vi "PH_uOPA_DelayController.PC Get data.vi"(0 "i ref in":refnum<vi>, 5 "error IO":errorcluster) -> (14 "i ref out":refnum<vi>, 19 "error out":errorcluster)   [LabVIEW 2014, in "PH_uOPA_DelayController.lvlib"]
doc: "This is the proc case \"Get Data\": It communicates with hardware to get data and writes them to own attributes."
uses:
  PH_uOPA_DelayController.lvlib
  PH_Basics/PH_StatusHandler/PH_StatusHandler.Status.ctl
  PH_Devices/PH_TKTDS-30xx/PH_TKTDS-30xx.Waveform to fetch.ctl
  PH_Devices/PH_TKTDS-30xx/PH_TKTDS-30xx.Waveform Limits.ctl
  PH_Devices/PH_TKTDS-30xx/PH_TKTDS-30xx.lvlib
  PH_Basics/PH_StatusHandler/PH_StatusHandler.lvlib
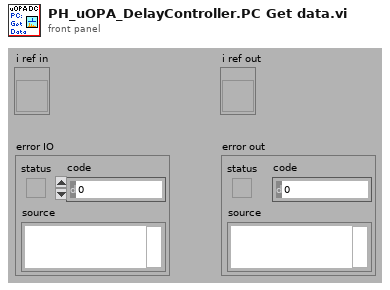
[diagram p1: front panel]
types:
  T1 = typedef "PH_StatusHandler.lvlib/PH_StatusHandler.Status.ctl" = i16
  T2 = typedef "PH_TKTDS-30xx.lvlib/PH_TKTDS-30xx.i attribute.ctl" = cluster{"Default VISA Resource":string, "VISA Resource Name":refnum<visa-resource-name>, "Revision":cluster{"Instrument Driver":string, "Instrument Firmware":string}, "Selftest":cluster{"Result":u32, "Message":string}, "Channels":T3[], "Trigger Configuration":T5, "Acquisition Configuration":T6, "Fetched Waveforms":T7[], "GUI Refs":T8, "State":T1, "Error Message":string, "Allow Prdc Loop?":bool}
  T3 = typedef "PH_TKTDS-30xx.lvlib/PH_TKTDS-30xx.Channel Config.ctl" = cluster{"Channel Name":string, "Input Impedance":string, "Max Input Frequency":string, "Vertical Coupling":i32, "Channel Enabled":bool, "Probe Attenuation":dbl, "Vertical Range":dbl, "Vertical Offset":dbl, "Waveform Limits":T4}
  T4 = typedef "PH_TKTDS-30xx.lvlib/PH_TKTDS-30xx.Waveform Limits.ctl" = cluster{"Start":i32, "End":i32}
  T5 = typedef "PH_TKTDS-30xx.lvlib/PH_TKTDS-30xx.Trigger Config.ctl" = cluster{"Source":string, "Slope":i32, "Level [V]":dbl}
  T6 = typedef "PH_TKTDS-30xx.lvlib/PH_TKTDS-30xx.Acquisition Config.ctl" = cluster{"Time base":dbl, "Record Length":u16, "Start Time":dbl, "Type":i32, "Continuous":bool}
  T7 = typedef "PH_TKTDS-30xx.lvlib/PH_TKTDS-30xx.fetched Waveform.ctl" = cluster{"Source":string, "Actual Points":u32, "Initial X":dbl, "X Increment":dbl, "Waveform Array":dbl[]}
  T8 = typedef "PH_TKTDS-30xx.lvlib/PH_TKTDS-30xx.GUI Refs.ctl" = cluster{"Trigger":refnum<vi>, "Acquisition":refnum<vi>, "State":refnum<vi>, "Delete":refnum<vi>, "Channel to be positioned":refnum<vi>, "Postion":refnum<vi>, "Display Intensity":refnum<vi>, "VISA Resource":refnum<vi>, "Channels":refnum<vi>[], "Graphs":refnum<vi>[]}
  T9 = typedef "PH_TKTDS-30xx.lvlib/PH_TKTDS-30xx.Waveform to fetch.ctl" = cluster{"Source":string, "Waveform Limits":T4}
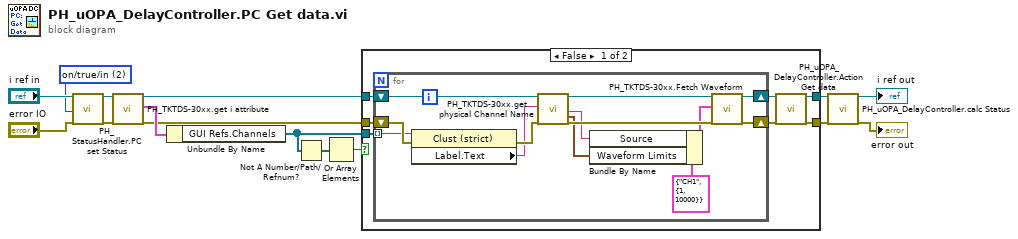
[diagram p0: block diagram]
diagram:
  w3 = T1 2 items=["no info", "off/false/out", "on/true/in", "Failure", "Alarm", "Status 1", "Status 2", "Status 3"] ("Status")
  n1 = call "PH_StatusHandler.PC set Status.vi"("i ref in"="i ref in", "Status"=w3, "error in (no error)"="error IO") -> ("i ref out"=w2:refnum<vi>, "error out"=w1:errorcluster)  [unwired: 15 in]
  n2 = call "PH_TKTDS-30xx.get i attribute.vi"("i ref in"=w2, "error in (no error)"=w1) -> ("i ref out"=w6:refnum<vi>, "i attribute"=w11:T2, "error out"=w7:errorcluster)  [unwired: 15 in]
  n3 = Unbundle By Name(w11) -> ("GUI Refs.Channels"=w8:refnum<vi>[])
  n4 = Not A Number/Path/Refnum?(number/path/refnum=w8) -> (NaN/Path/Refnum?=w10:bool[])
  n5 = Or Array Elements(Boolean array=w10) -> (logical OR=w9:bool)
  n6 = case shown="False" w9 {
    tunnel: [w20 w37] -> w5
    tunnel: [w19 w36] -> w4
    tunnel: w8 -> [w18 _]
    tunnel: w6 -> [w17 w37]
    tunnel: w7 -> [w16 w36]
    frame False {
      n7 = for {
        shift-right: [w33] -> w21
        shift-left: w16 -> [w32]
        shift-right: [w34] -> w22
        shift-left: w17 -> [w35]
        tunnel: w18 -> [w30] mode=indexing
        n8 = property class="Clust (strict)"(reference=w30, error in=w32) -> (error out=w31:errorcluster, "Label.Text"=w29:string)  [unwired: 1 out]
        n9 = call "PH_TKTDS-30xx.get physical Channel Name.vi"("i ref in"=w35, "GUI Element Name"=w29, "error in"=w31) -> ("i ref out"=w27:refnum<vi>, "Physical Channel Name"=w25:string, "Waveform Limits"=w24:T4, "error out"=w28:errorcluster)  [unwired: 13 in]
        n10 = Bundle By Name(cluster=T9 {"Source"="CH1", "Waveform Limits"={"Start"=1, "End"=10000}} ("Waveform to fetch"), "Source"=w25, "Waveform Limits"=w24) -> (w26:T9)
        n11 = call "PH_TKTDS-30xx.Fetch Waveform.vi"("i ref in"=w27, "Waveform to fetch"=w26, "error IO"=w28) -> ("i ref out"=w34:refnum<vi>, "error out"=w33:errorcluster)  [unwired: 15 in]
      }
      n12 = call "PH_uOPA_DelayController.Action Get data.vi"("i ref in"=w22, "error IO"=w21) -> ("i ref out"=w20:refnum<vi>, "error out"=w19:errorcluster)  [unwired: 16 in]
    }
    frame True {
    }
  }
  n13 = call "PH_uOPA_DelayController.calc Status.vi"("i ref in"=w5, "error in"=w4) -> ("i ref out"=→"i ref out":refnum<vi>, "error out"=→"error out":errorcluster)  [unwired: 16 in]
